vi "Select Panther Scan File to load.vi"(11 "PantherScan bin Files":path[](array[path])) -> (2 "Continue?":bool, 3 "Panther Scan Selected":path)   [LabVIEW 2019, in "Panther Dashboard.lvlib"]
uses:
  Panther Dashboard.lvlib
panel:
  in  "Panther Scans":i32(listbox)
  # "Panther Dashboard saves a binary file\nfor each scanned target next to the\nLabVIEW Project with the following format\n\n<LabVIEW Project folder Path>\\PantherScan.[Target].bin\n\nChoose the scanned target you'd like to work with.\n\n\nTip:\nYou can track PantherScan binary files using source code\ncontrol, you'll need to make sure all the Developers have the\nsame project path on their computers, example:\n\nDeveloper 1:\nC:\\GitClones\\<Project Path>\n\nDeveloper 2:\nC:\\GitClones\\<Project Path>"
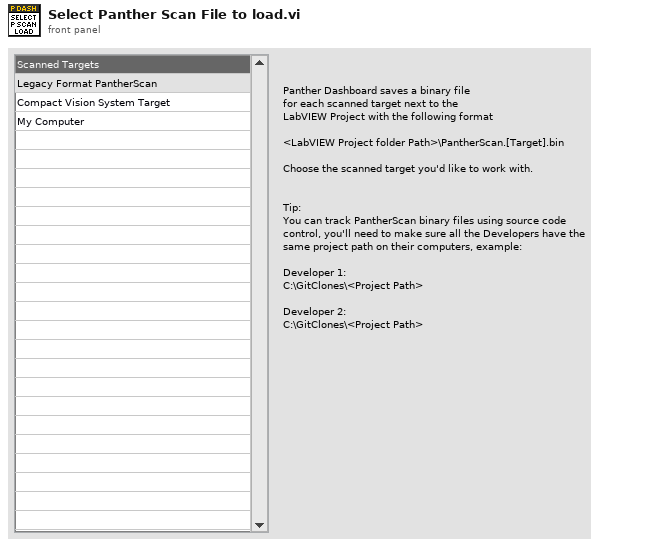
[diagram p1: front panel]
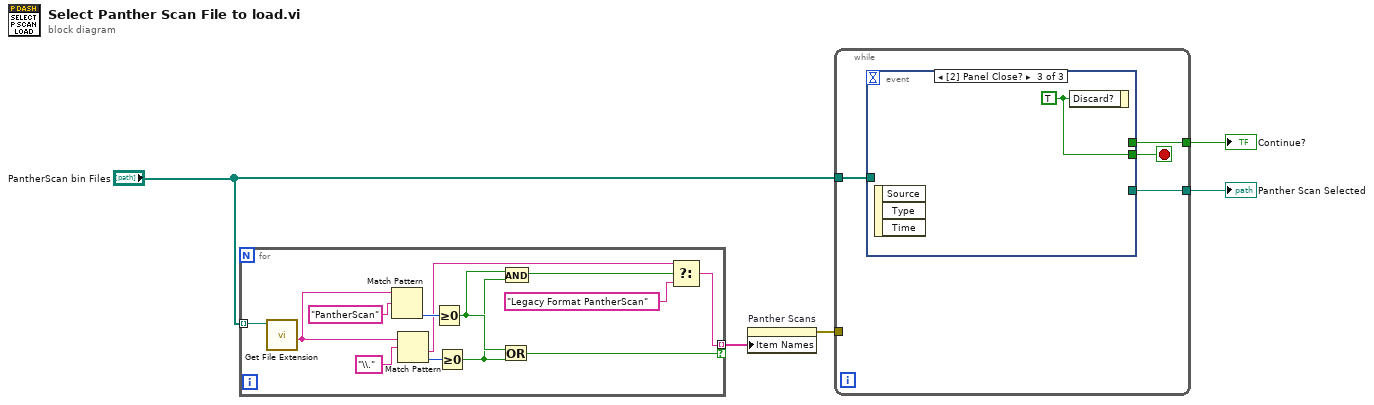
[diagram p0: block diagram]
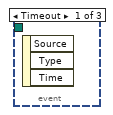
[diagram p2: hidden frame]
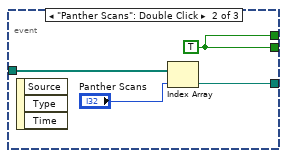
[diagram p3: hidden frame]
diagram:
  n1 = for {
    tunnel: [w13] -> w1 mode=indexing if=w8
    tunnel: "PantherScan bin Files" -> [w18] mode=indexing
    n2 = call <vilib>:"Get File Extension.vi"("file"=w18) -> ("filename without extension"=w7:string)  [unwired: 6 in, 4 out]
    n3 = Match Pattern(string=w7, regular expression="PantherScan") -> (offset past match=w14:i32)  [unwired: 1 in, 3 out]
    n4 = Match Pattern(string=w7, regular expression="\\.") -> (after substring=w11:string, offset past match=w16:i32)  [unwired: 1 in, 2 out]
    n5 = Greater Or Equal To 0?(x=w14) -> (x >= 0?=w10:bool)
    n6 = Greater Or Equal To 0?(x=w16) -> (x >= 0?=w9:bool)
    n7 = Or(x=w10, y=w9) -> (x .or. y?=w8:bool)
    n8 = And(x=w10, y=w9) -> (x .and. y?=w12:bool)
    n9 = Select(t=w11, s=w12, f="Legacy Format PantherScan") -> (s? t:f=w13:string)
  }
  n10 = property on="Panther Scans" class="LstBox (strict)"("Item Names"=w1) -> (error out=w5:errorcluster)  [unwired: 2 in, 1 out]
  n11 = while {
    tunnel: "PantherScan bin Files" -> [w21]
    tunnel: [w20] -> w4
    tunnel: w5 -> [_]
    tunnel: [w19] -> w2
    stop <- w22 stop-if-true
    n12 = event shown="[2] Panel Close?" {
      selector: _ -> [_ _ _]
      dyn-events: _ -> [_ _ _]
      timeout: _ -> [_ _ _]
      tunnel: [_ w23 w27] -> w22
      tunnel: w21 -> [_ w25 _]
      tunnel: [_ w24 _] -> w20
      tunnel: [_ w23 _] -> w19
      event Timeout {
        n13 = event-data() -> ()  [unwired: 1 in, 3 out]
      }
      event "Panther Scans": Double Click {
        w23 = TRUE ("Discard?")
        n14 = event-data() -> ()  [unwired: 1 in, 3 out]
        n15 = Index Array(array=w25, index="Panther Scans") -> (element=w24:path)
      }
      event Panel Close? {
        w27 = TRUE ("Discard?")
        n16 = event-data() -> ()  [unwired: 1 in, 3 out]
        n17 = event-data("Discard?"=w27) -> ()  [unwired: 1 in, 1 out]
      }
    }
  }
  "Continue?" <- w2
  "Panther Scan Selected" <- w4
